vi "pH电极校准.vi"() -> ()   [LabVIEW 2016, in "国弘多参数.lvlib"]
uses:
  <vilib>/Analysis/NI_AALBase.lvlib
panel:
  out "当前检测值":dbl
  out "提示":string
  in  "第二点通过校正":bool
  in  "第一点通过校正":bool
  in  "第二点校正":bool
  in  "第一点校正":bool
  out "标液2":dbl
  out "标液1":dbl
  out "当前信号值":dbl
  out "偏移值补偿":dbl
  out "电极斜率":dbl
  out "电极零点":dbl
  # "酸碱度电极设定"
  # "mV"
  # "pH"
  # "%"
  # "mV"
  # "电极校正"
  # "标准液值:"
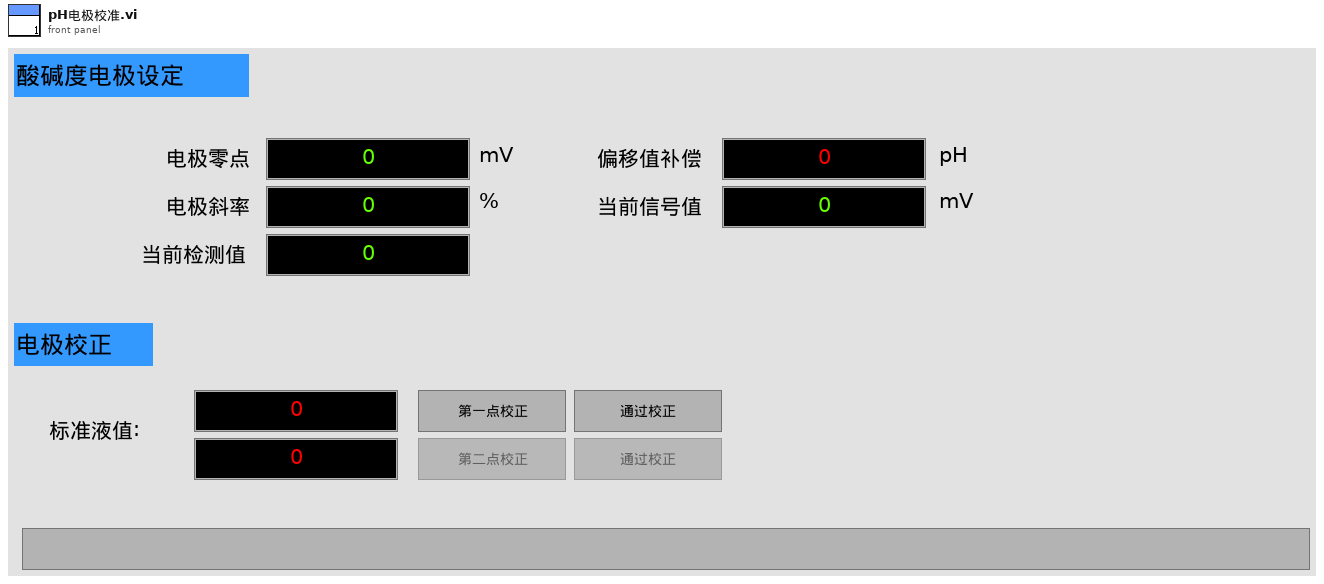
[diagram p1: front panel]
types:
  T1 = typedef "国弘多参数.lvlib/校准步骤.ctl" = enum16{"待机", "第一点校准启动", "第二点校准启动", "第一点校准写入", "第二点校准写入", "第一点校准失败", "第二点校准失败"}
  T2 = enum8{"Enabled", "Disabled", "Disabled and Grayed Out"}
  T3 = cluster{"电极状态标志":u16, "电极型号标志":u16, "酸碱度测量值":sgl, "温度测量值":sgl, "酸碱度信号值":sgl, "温度信号值":sgl, "酸碱度偏移修正值":sgl, "温度偏移修正值":sgl, "手动温度补偿值":sgl, "酸碱度电极零点":sgl, "酸碱度电极斜率":sgl, "第1点标准值记录":sgl, "第1点信号值记录":sgl, "第1点温度值记录":sgl, "第2点标准值记录":sgl, "第2点信号值记录":sgl, "第2点温度值记录":sgl, "命令滤波设定":u16, "温度模式":enum16{"ATC", "MTC"}, "生产批次":u16, "电极序号":u16, "串口地址":u16, "串口波特率":enum16{"9600", "19200", "115200"}, "串口校验位":enum16{"NONE", "ODD", "EVEN"}, "串口停止位":enum16{"1bit", "2bit"}, "第一点标准值":sgl, "第二点标准值":sgl}
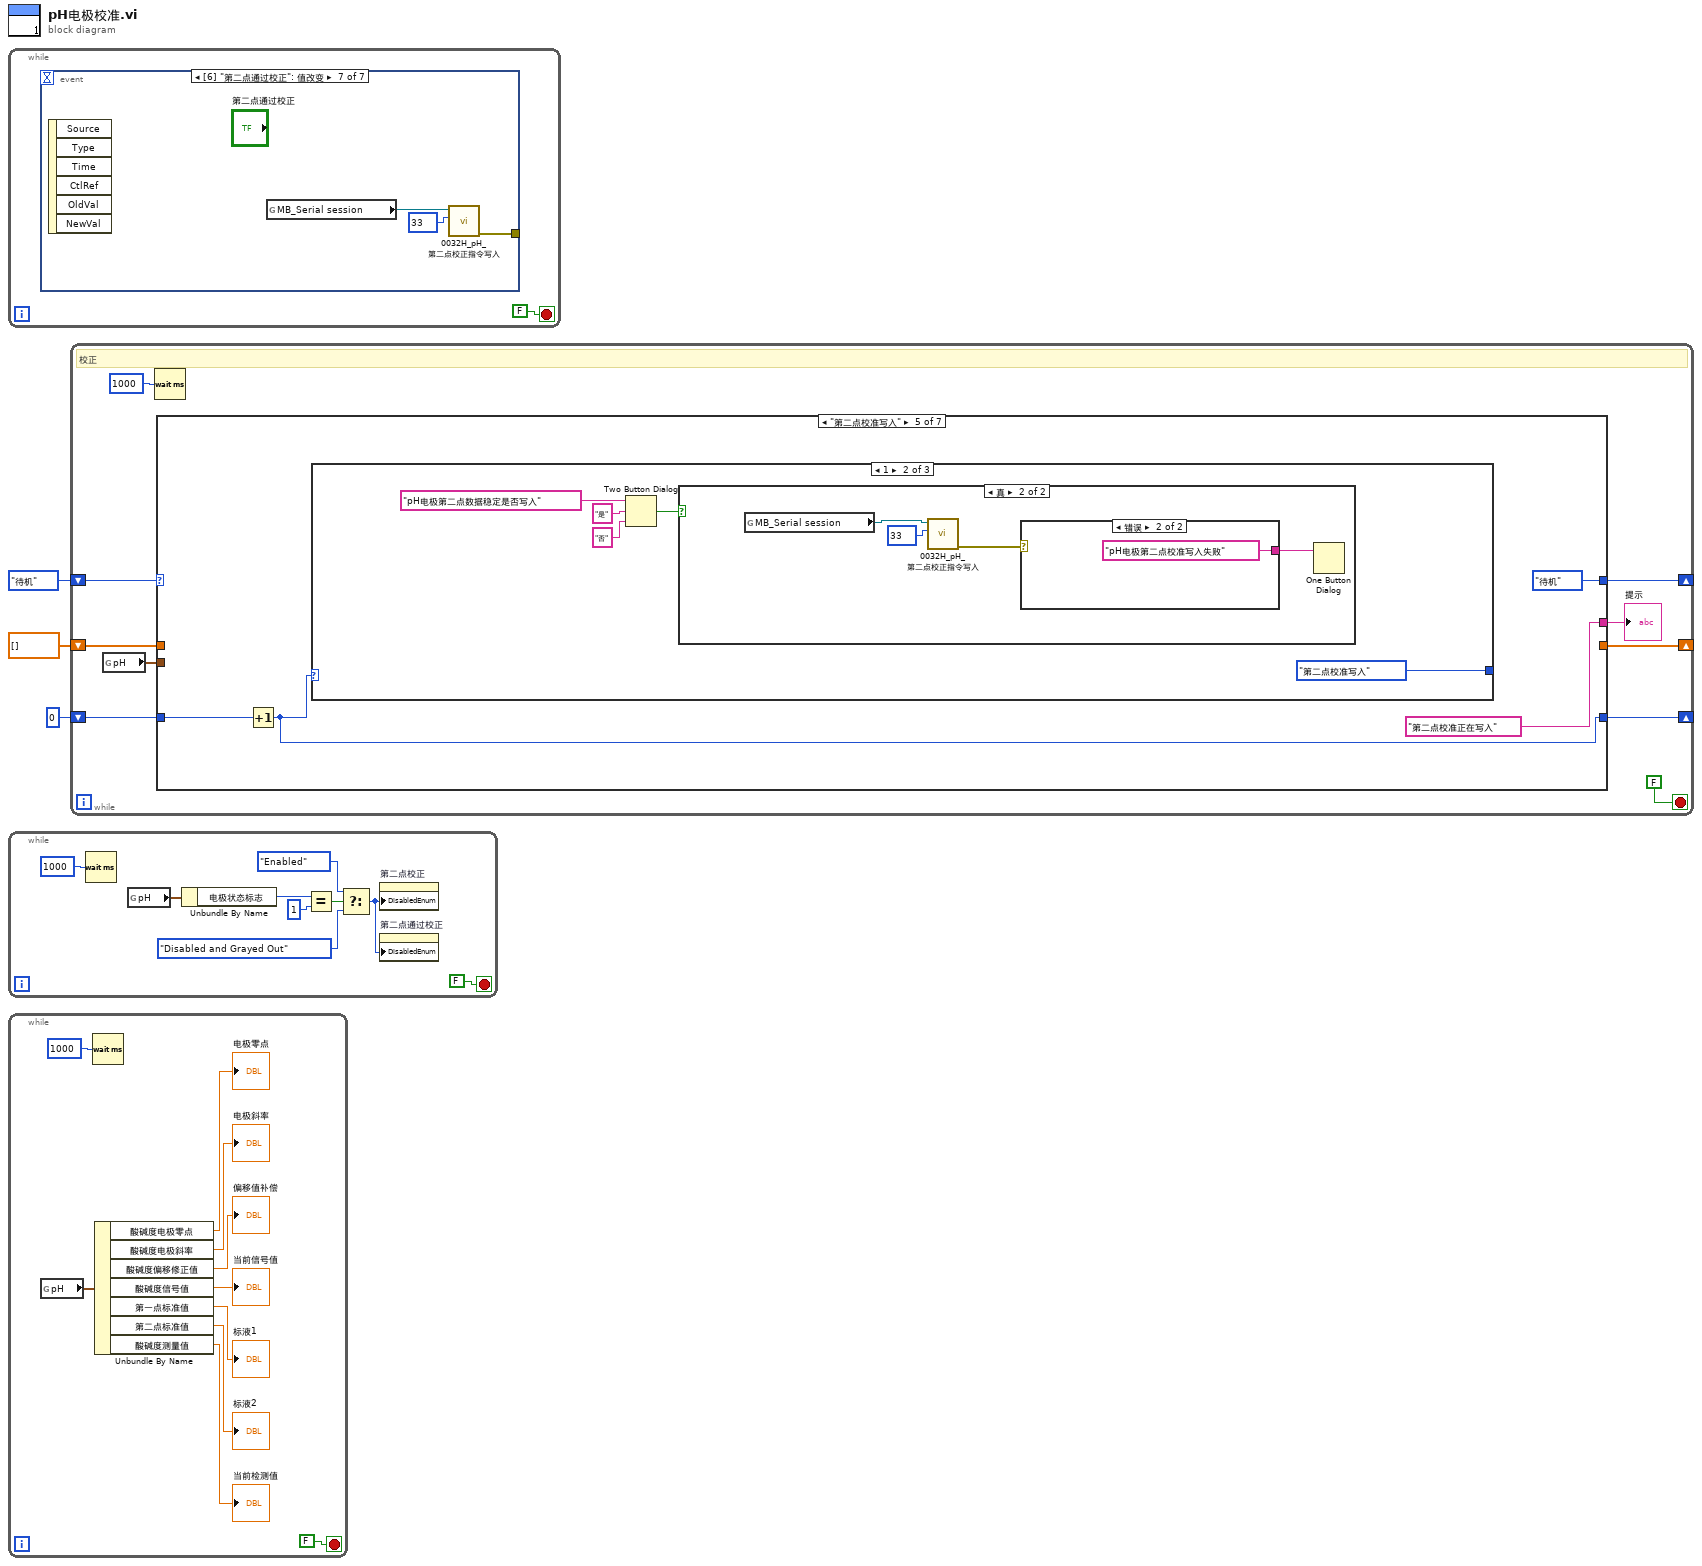
[diagram p0: block diagram]
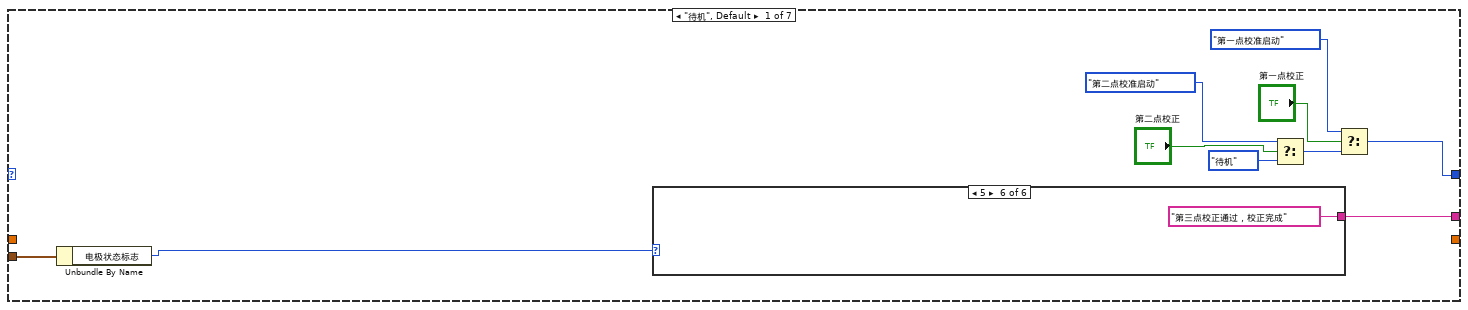
[diagram p2: hidden frame]
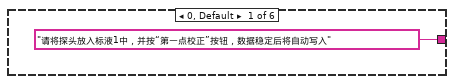
[diagram p3: hidden frame]
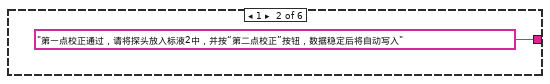
[diagram p4: hidden frame]
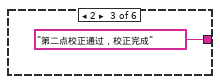
[diagram p5: hidden frame]
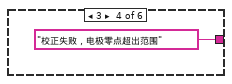
[diagram p6: hidden frame]
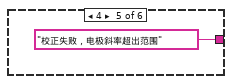
[diagram p7: hidden frame]
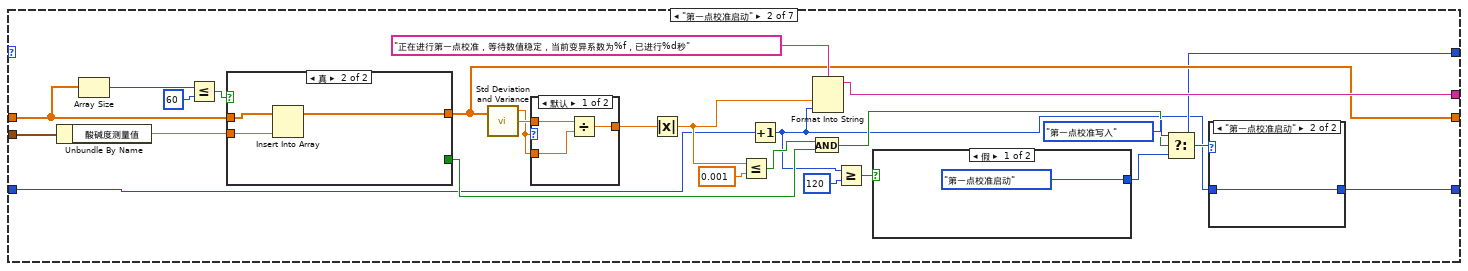
[diagram p8: hidden frame]
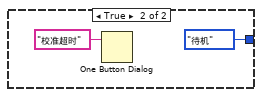
[diagram p11: hidden frame]
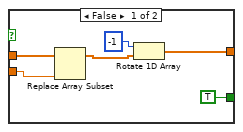
[diagram p12: hidden frame]
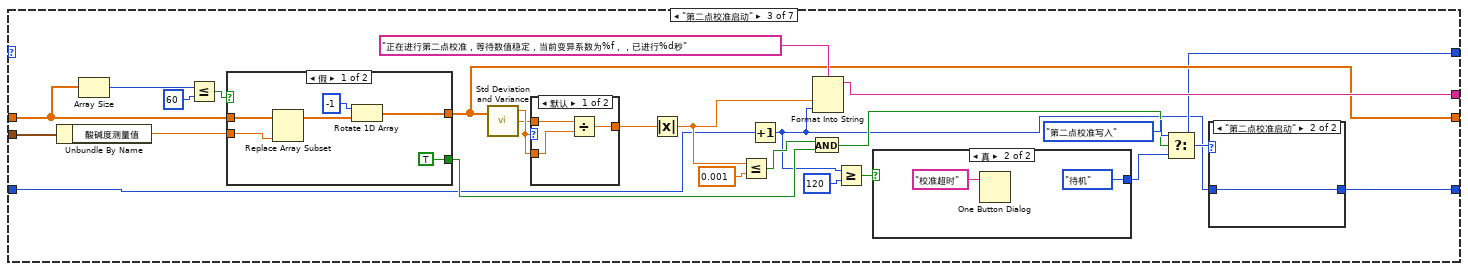
[diagram p13: hidden frame]
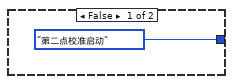
[diagram p16: hidden frame]
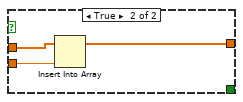
[diagram p17: hidden frame]
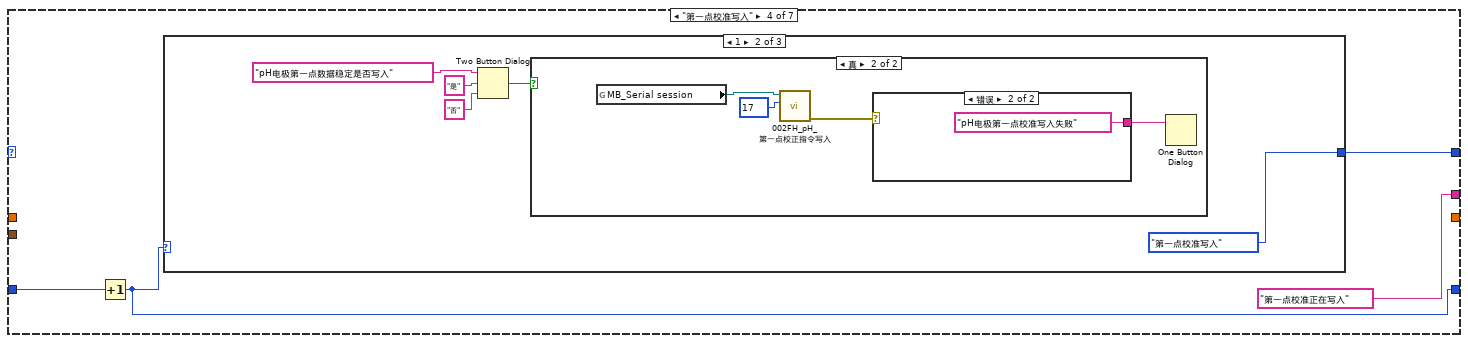
[diagram p18: hidden frame]
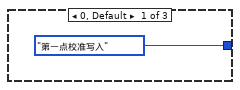
[diagram p19: hidden frame]
diagram:
  n1 = while {
    stop <- FALSE stop-if-true
    n2 = event shown="[6] \"第二点通过校正\": 值改变" {
      selector: _ -> [_ _ _ _ _ _ _]
      dyn-events: _ -> [_ _ _ _ _ _ _]
      timeout: _ -> [_ _ _ _ _ _ _]
      tunnel: [_ _ w9 w12 w15 w18 w21] -> _
      event Timeout {
        n3 = event-data() -> ()  [unwired: 1 in, 3 out]
      }
      event "标液1", "标液2", "偏移值补偿": Mouse Down {
        n4 = event-data() -> ("CtlRef"=w8:refnum<vi>)  [unwired: 1 in, 7 out]
        n5 = property class="DigNum (严格)"(reference=w8) -> (reference out=w5:refnum<vi>, "Value"=w6:dbl)  [unwired: 1 in, 1 out]
        n6 = call "数字键盘.vi"("OldNumber"=w6) -> ("NewNumber"=w7:sgl)
        n7 = property class="DigNum (严格)"(reference=w5, "Val(Sgnl)"=w7) -> ()  [unwired: 1 in, 2 out]
      }
      event "偏移值补偿": Value Change {
        n8 = event-data() -> ("NewVal"=w11:dbl)  [unwired: 1 in, 5 out]
        n9 = global read "过程全局变量.vi" "MB_Serial session"() -> (w10:refnum<class "MB_Master_Serial.lvclass">)
        n10 = call "000CH_pH_pH偏移修正值写入.vi"("数值"=w11, "MB_Serial session in"=w10) -> ("error out"=w9:errorcluster)  [unwired: 8 in, 1 out]
      }
      event "标液1": Value Change {
        n11 = event-data() -> ("NewVal"=w13:dbl)  [unwired: 1 in, 5 out]
        n12 = global read "过程全局变量.vi" "MB_Serial session"() -> (w14:refnum<class "MB_Master_Serial.lvclass">)
        n13 = call "0030H_pH_第一点标准值写入.vi"("数值"=w13, "MB_Serial session in"=w14) -> ("error out"=w12:errorcluster)  [unwired: 8 in, 1 out]
      }
      event "标液2": Value Change {
        n14 = event-data() -> ("NewVal"=w16:dbl)  [unwired: 1 in, 5 out]
        n15 = global read "过程全局变量.vi" "MB_Serial session"() -> (w17:refnum<class "MB_Master_Serial.lvclass">)
        n16 = call "0033H_pH_第二点标准值写入.vi"("数值"=w16, "MB_Serial session in"=w17) -> ("error out"=w15:errorcluster)  [unwired: 8 in, 1 out]
      }
      event "第一点通过校正": Value Change {
        n17 = event-data() -> ()  [unwired: 1 in, 6 out]
        n18 = global read "过程全局变量.vi" "MB_Serial session"() -> (w20:refnum<class "MB_Master_Serial.lvclass">)
        n19 = call "002FH_pH_第一点校正指令写入.vi"("数值"=u16 17, "MB_Serial session in"=w20) -> ("error out"=w18:errorcluster)  [unwired: 8 in, 1 out]
      }
      event "第二点通过校正": Value Change {
        n20 = event-data() -> ()  [unwired: 1 in, 6 out]
        n21 = global read "过程全局变量.vi" "MB_Serial session"() -> (w23:refnum<class "MB_Master_Serial.lvclass">)
        n22 = call "0032H_pH_第二点校正指令写入.vi"("数值"=u16 33, "MB_Serial session in"=w23) -> ("error out"=w21:errorcluster)  [unwired: 8 in, 1 out]
      }
    }
  }
  n23 = while {
    stop <- FALSE stop-if-true
    n24 = Wait (ms)(milliseconds to wait=u32 1000 ("等待时间（毫秒）")) -> ()  [unwired: 1 out]
    n25 = global read "过程全局变量.vi" "pH"() -> (w30:T3)
    n26 = Unbundle By Name(w30) -> ("电极状态标志"=w29:u16)
    n27 = Equal?(x=w29, y=u16 1) -> (x = y?=w24:bool)
    n28 = Select(t=T2."Enabled" ("禁用"), s=w24, f=T2."Disabled and Grayed Out" ("禁用")) -> (s? t:f=w25:T2)
    n29 = property on="第二点校正" class="Bool"("DisabledEnum"=w25) -> ()  [unwired: 2 in, 2 out]
    n30 = property on="第二点通过校正" class="Bool"("DisabledEnum"=w25) -> ()  [unwired: 2 in, 2 out]
  }
  n31 = while {
    stop <- FALSE stop-if-true
    n32 = global read "过程全局变量.vi" "pH"() -> (w40:T3)
    n33 = Wait (ms)(milliseconds to wait=u32 1000 ("等待时间（毫秒）")) -> ()  [unwired: 1 out]
    n34 = Unbundle By Name(w40) -> ("酸碱度电极零点"=→"电极零点":sgl, "酸碱度电极斜率"=→"电极斜率":sgl, "酸碱度偏移修正值"=→"偏移值补偿":sgl, "酸碱度信号值"=→"当前信号值":sgl, "第一点标准值"=→"标液1":sgl, "第二点标准值"=→"标液2":sgl, "酸碱度测量值"=→"当前检测值":sgl)
  }
  n35 = while "While循环" {
    shift-right: [w51] -> _
    shift-left: 校准步骤."待机" ("枚举") -> [w52]
    shift-right: [w45] -> _
    shift-left: sgl[] [] -> [w46]
    shift-right: [w43] -> _
    shift-left: 0 -> [w44]
    stop <- FALSE stop-if-true
    # "校正"
    n36 = global read "过程全局变量.vi" "pH"() -> (w48:T3)
    n37 = Wait (ms)(milliseconds to wait=u32 1000 ("等待时间（毫秒）")) -> ()  [unwired: 1 out]
    n38 = case shown="\"第二点校准写入\"" w52 {
      tunnel: [w60 w72 w115 w151 校准步骤."待机" ("枚举") 校准步骤."待机" ("枚举") 校准步骤."待机" ("枚举")] -> w51
      tunnel: [w58 w86 w123 "第一点校准正在写入" ("提示") "第二点校准正在写入" ("提示") "第一点校准失败" ("提示") "第二点校准失败" ("提示")] -> w49
      tunnel: w48 -> [w57 w93 w124 _ _ _ _]
      tunnel: w46 -> [_ w79 w122 _ _ _ _]
      tunnel: [_ w78 w121 _ _ _ _] -> w45
      tunnel: w44 -> [_ w76 w119 w153 w169 w186 w191]
      tunnel: [_ w70 w113 w152 w168 w185 w190] -> w43
      frame "待机", Default {
        n39 = Unbundle By Name(w57) -> ("电极状态标志"=w59:u16)
        n40 = case shown="5" w59 {
          tunnel: ["请将探头放入标液1中，并按“第一点校正”按钮，数据稳定后将自动写入" ("提示") "第一点校正通过，请将探头放入标液2中，并按“第二点校正”按钮，数据稳定后将自动写入" ("提示") "第二点校正通过，校正完成" ("提示") "校正失败，电极零点超出范围" ("提示") "校正失败，电极斜率超出范围" ("提示") "第三点校正通过，校正完成" ("提示")] -> w58
          frame 0, Default {
          }
          frame 1 {
          }
          frame 2 {
          }
          frame 3 {
          }
          frame 4 {
          }
          frame 5 {
          }
        }
        n41 = Select(t=校准步骤."第二点校准启动" ("枚举"), s="第二点校正", f=校准步骤."待机" ("枚举")) -> (s? t:f=w53:T1)
        n42 = Select(t=校准步骤."第一点校准启动" ("枚举"), s="第一点校正", f=w53) -> (s? t:f=w60:T1)
      }
      frame "第一点校准启动" {
        n43 = Unbundle By Name(w93) -> ("酸碱度测量值"=w89:sgl)
        n44 = Array Size(array=w79) -> (size(s)=w92:i32)
        n45 = Less Or Equal?(x=w92, y=60) -> (x <= y?=w90:bool)
        n46 = case shown="真" w90 {
          tunnel: w79 -> [w106 w109]
          tunnel: w89 -> [w104 w108]
          tunnel: [w102 w107] -> w78
          tunnel: [TRUE _] -> w82
          frame False {
            n47 = Replace Array Subset(array=w106, new element=w104) -> (w105:sgl[])  [unwired: 1 in]
            n48 = Rotate 1D Array(1:w105, 2:-1 ("n")) -> (0:w102:sgl[])
          }
          frame True {
            n49 = Insert Into Array(array=w109, new element=w108) -> (w107:sgl[])  [unwired: 1 in]
          }
        }
        n50 = call <vilib>:"Std Deviation and Variance.vi"("X"=w78) -> ("mean"=w69:dbl, "standard deviation"=w88:dbl)  [unwired: 1 in, 1 out]
        n51 = case shown="默认" w69 {
          tunnel: w88 -> [w96 _]
          tunnel: [w95 _] -> w85
          tunnel: w69 -> [w94 _]
          frame Default {
            n52 = Divide(x=w96, y=w94) -> (x/y=w95:dbl)
          }
          frame 0 {
          }
        }
        n53 = Absolute Value(x=w85) -> (abs(x)=w77:dbl)
        n54 = Less Or Equal?(x=w77, y=0.001) -> (x <= y?=w81:bool)
        n55 = Increment(x=w76) -> (x+1=w71:i32)
        n56 = And(x=w81, y=w82) -> (x .and. y?=w80:bool)
        n57 = Format Into String(format string="正在进行第一点校准，等待数值稳定，当前变异系数为%f，已进行%d秒" ("格式字符串"), w77, w71) -> (resulting string=w86:string)  [unwired: 2 in, 1 out]
        n58 = Greater Or Equal?(x=w71, y=120) -> (x >= y?=w74:bool)
        n59 = case shown="假" w74 {
          tunnel: [校准步骤."第一点校准启动" ("枚举") 校准步骤."待机" ("枚举")] -> w73
          frame False {
          }
          frame True {
            n60 = One Button Dialog(message="校准超时" ("消息")) -> ()  [unwired: 1 in, 1 out]
          }
        }
        n61 = Select(t=校准步骤."第一点校准写入" ("枚举"), s=w80, f=w73) -> (s? t:f=w72:T1)
        n62 = case shown="\"第一点校准启动\"" w72 {
          tunnel: w71 -> [_ w97]
          tunnel: [_ w97] -> w70
          frame "待机", Default {
          }
          frame "第一点校准启动" {
          }
        }
      }
      frame "第二点校准启动" {
        n63 = Unbundle By Name(w124) -> ("酸碱度测量值"=w131:sgl)
        n64 = Array Size(array=w122) -> (size(s)=w134:i32)
        n65 = Less Or Equal?(x=w134, y=60) -> (x <= y?=w132:bool)
        n66 = case shown="假" w132 {
          tunnel: w122 -> [w147 w150]
          tunnel: w131 -> [w145 w149]
          tunnel: [w143 w148] -> w121
          tunnel: [TRUE _] -> w127
          frame False {
            n67 = Replace Array Subset(array=w147, new element=w145) -> (w146:sgl[])  [unwired: 1 in]
            n68 = Rotate 1D Array(1:w146, 2:-1 ("n")) -> (0:w143:sgl[])
          }
          frame True {
            n69 = Insert Into Array(array=w150, new element=w149) -> (w148:sgl[])  [unwired: 1 in]
          }
        }
        n70 = call <vilib>:"Std Deviation and Variance.vi"("X"=w121) -> ("mean"=w111:dbl, "standard deviation"=w110:dbl)  [unwired: 1 in, 1 out]
        n71 = case shown="默认" w111 {
          tunnel: [w137 _] -> w112
          tunnel: w111 -> [w136 _]
          tunnel: w110 -> [w135 _]
          frame Default {
            n72 = Divide(x=w135, y=w136) -> (x/y=w137:dbl)
          }
          frame 0 {
          }
        }
        n73 = Absolute Value(x=w112) -> (abs(x)=w120:dbl)
        n74 = Less Or Equal?(x=w120, y=0.001) -> (x <= y?=w126:bool)
        n75 = Increment(x=w119) -> (x+1=w114:i32)
        n76 = And(x=w126, y=w127) -> (x .and. y?=w125:bool)
        n77 = Format Into String(format string="正在进行第二点校准，等待数值稳定，当前变异系数为%f，，已进行%d秒" ("格式字符串"), w120, w114) -> (resulting string=w123:string)  [unwired: 2 in, 1 out]
        n78 = Greater Or Equal?(x=w114, y=120) -> (x >= y?=w117:bool)
        n79 = case shown="真" w117 {
          tunnel: [校准步骤."第二点校准启动" ("枚举") 校准步骤."待机" ("枚举")] -> w116
          frame False {
          }
          frame True {
            n80 = One Button Dialog(message="校准超时" ("消息")) -> ()  [unwired: 1 in, 1 out]
          }
        }
        n81 = Select(t=校准步骤."第二点校准写入" ("枚举"), s=w125, f=w116) -> (s? t:f=w115:T1)
        n82 = case shown="\"第二点校准启动\"" w115 {
          tunnel: w114 -> [_ w138]
          tunnel: [_ w138] -> w113
          frame "待机", Default {
          }
          frame "第二点校准启动" {
          }
        }
      }
      frame "第一点校准写入" {
        n83 = Increment(x=w153) -> (x+1=w152:i32)
        n84 = case shown="1" w152 {
          tunnel: [校准步骤."第一点校准写入" ("枚举") 校准步骤."第一点校准写入" ("枚举") 校准步骤."待机" ("枚举")] -> w151
          frame 0, Default {
          }
          frame 1 {
            n85 = Two Button Dialog(message="pH电极第一点数据稳定是否写入" ("消息"), 1:"否" ("F按钮名称（“取消”）"), 2:"是" ("T按钮名称（“确定”）")) -> (T button?=w156:bool)
            n86 = case shown="真" w156 {
              frame False {
              }
              frame True {
                n87 = global read "过程全局变量.vi" "MB_Serial session"() -> (w163:refnum<class "MB_Master_Serial.lvclass">)
                n88 = call "002FH_pH_第一点校正指令写入.vi"("数值"=u16 17, "MB_Serial session in"=w163) -> ("error out"=w161:errorcluster)  [unwired: 8 in, 1 out]
                n89 = case shown="错误" w161 {
                  tunnel: ["pH电极第一点校准写入成功" ("消息") "pH电极第一点校准写入失败" ("消息")] -> w162
                  frame No Error {
                  }
                  frame Error {
                  }
                }
                n90 = One Button Dialog(message=w162) -> ()  [unwired: 1 in, 1 out]
              }
            }
          }
          frame 2 {
          }
        }
      }
      frame "第二点校准写入" {
        n91 = Increment(x=w169) -> (x+1=w168:i32)
        n92 = case shown="1" w168 {
          tunnel: [校准步骤."第二点校准写入" ("枚举") 校准步骤."第二点校准写入" ("枚举") 校准步骤."待机" ("枚举")] -> _
          frame 0, Default {
          }
          frame 1 {
            n93 = Two Button Dialog(message="pH电极第二点数据稳定是否写入" ("消息"), 1:"否" ("F按钮名称（“取消”）"), 2:"是" ("T按钮名称（“确定”）")) -> (T button?=w173:bool)
            n94 = case shown="真" w173 {
              frame False {
              }
              frame True {
                n95 = global read "过程全局变量.vi" "MB_Serial session"() -> (w181:refnum<class "MB_Master_Serial.lvclass">)
                n96 = call "0032H_pH_第二点校正指令写入.vi"("数值"=u16 33, "MB_Serial session in"=w181) -> ("error out"=w179:errorcluster)  [unwired: 8 in, 1 out]
                n97 = case shown="错误" w179 {
                  tunnel: ["pH电极第二点校准写入成功" ("消息") "pH电极第二点校准写入失败" ("消息")] -> w178
                  frame No Error {
                  }
                  frame Error {
                  }
                }
                n98 = One Button Dialog(message=w178) -> ()  [unwired: 1 in, 1 out]
              }
            }
          }
          frame 2 {
          }
        }
      }
      frame "第一点校准失败" {
        n99 = Two Button Dialog(message="第一点校准失败是否重新校准" ("消息")) -> ()  [unwired: 2 in, 1 out]
        n100 = Increment(x=w186) -> (x+1=w185:i32)
      }
      frame "第二点校准失败" {
        n101 = Increment(x=w191) -> (x+1=w190:i32)
      }
    }
    "提示" <- w49
  }
